vi "Serial_readV1.vi"() -> ()   [LabVIEW 2014]
uses:
  <vilib>/Instr/_visa.llb/VISA Set IO Buffer Mask.ctl
  <vilib>/Instr/_visa.llb/VISA Flush IO Buffer Mask.ctl
  <vilib>/Instr/_visa.llb/VISA Configure Serial Port (Instr).vi
panel:
  out "Svoris 2":cluster{dbl}(graph)
  out "Temperatura":cluster{dbl}(graph)
  in  "Nunulinti":bool
  out "Svoris, N":dbl format="%#_4f"
  out "Svoris":cluster{dbl}(graph)
  out "Svoris, N":dbl(slide) scale=0.0..10000.0
  out "Svoris":dbl
  in  "milliseconds to wait":u32=200
  out "Svoris":dbl(knob) scale=0.0..3.3
  in  "stop":bool
  in  "VISA resource name":refnum<visa-resource-name>
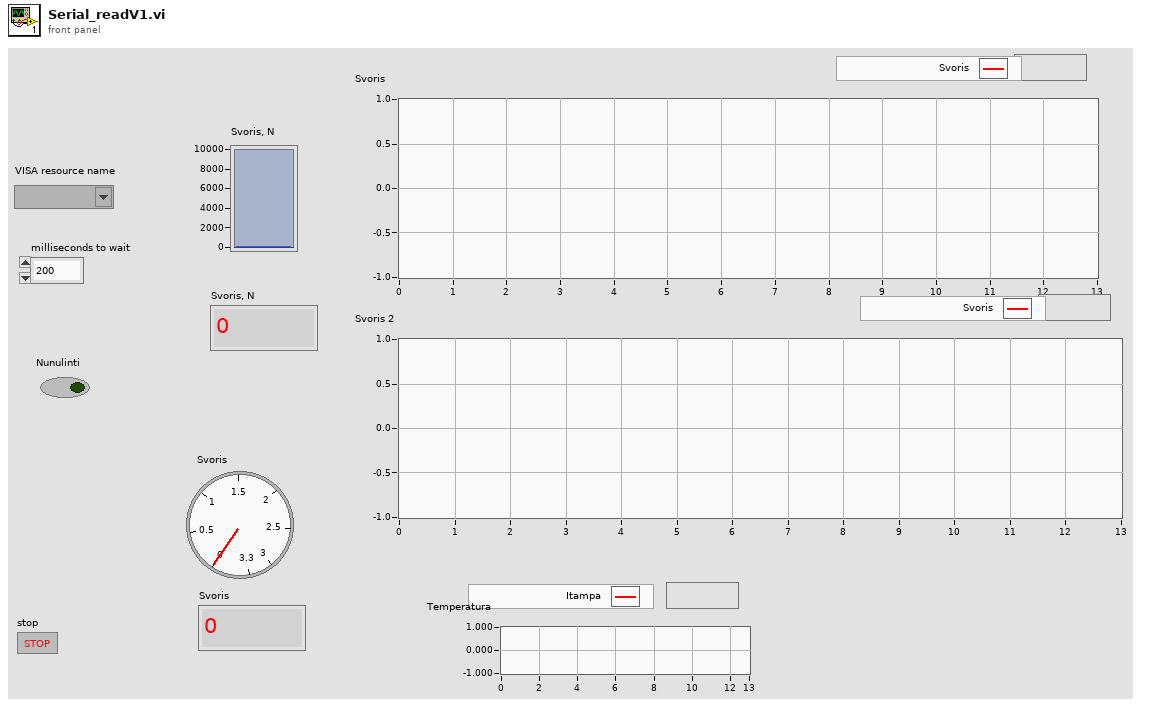
[diagram p1: front panel]
types:
  T1 = typedef "VISA Set IO Buffer Mask.ctl" = u16
  T2 = typedef "VISA Flush IO Buffer Mask.ctl" = u16
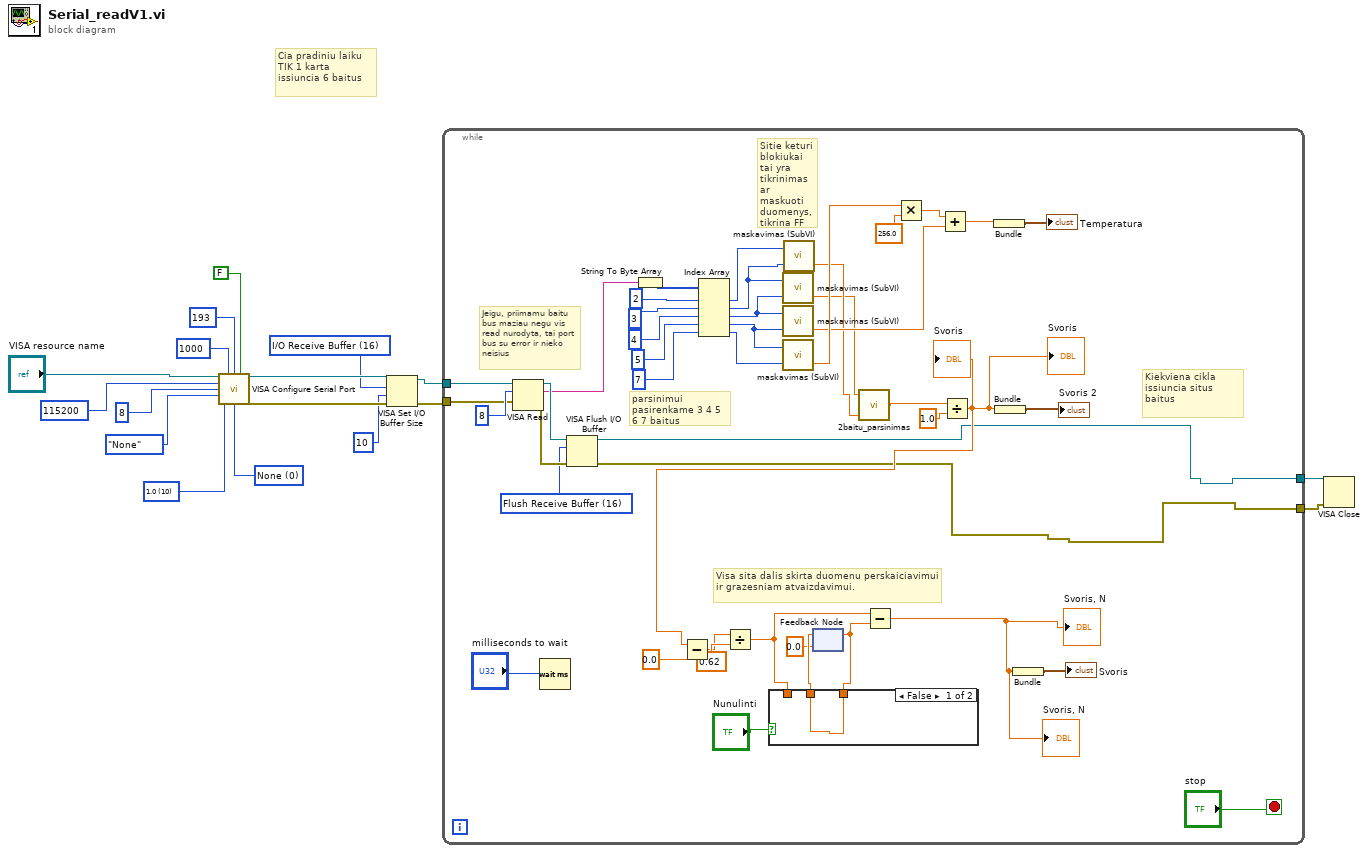
[diagram p0: block diagram]
diagram:
  w7 = T1 16 items=["I/O Receive Buffer"=16, "I/O Transmit Buffer"=32, "I/O Receive and Transmit Buffer"=48] ("Mask")
  w13 = u16 0 items=["None", "XON/XOFF", "RTS/CTS", "XON/XOFF & RTS/CTS", "DTR/DSR", "XON/XOFF & DTR/DSR"] ("flow control (0:none)")
  w14 = u16 10 items=["1.0"=10, "1.5"=15, "2.0"=20] ("stop bits (10: 1 bit)")
  # "Cia pradiniu laiku TIK 1 karta issiuncia 6 baitus"
  n1 = call-poly "VISA Configure Serial Port"("VISA resource name"="VISA resource name", "timeout (10sec)"=u32 1000, "termination char\n(0xA = '\\n' = LF)"=u8 193 ("termination char\n(0xA = '\\n' = LF)"), "Enable Termination\nChar (T)"=FALSE ("Enable Termination\nChar (T)"), "baud rate (9600)"=u32 115200, "data bits (8)"=u16 8, "parity (0:none)"=enum16{"None", "Odd", "Even", "Mark", "Space"}."None", "stop bits (10: 1 bit)"=w14, "flow control (0:none)"=w13) -> ("VISA resource name out"=w9:refnum<visa-resource-name>, "error out"=w10:errorcluster)  [unwired: 5 in]
  n2 = VISA Set I/O Buffer Size(VISA resource name=w9, mask (16)=w7, size (4096)=u32 10, error in (no error)=w10) -> (VISA resource name out=w3:refnum<visa-resource-name>, error out=w6:errorcluster)
  n3 = while {
    tunnel: w3 -> [w61]
    tunnel: w6 -> [w56]
    tunnel: [w19] -> w2
    tunnel: [w18] -> w1
    stop <- "stop" stop-if-true
    w51 = T2 16 items=["Flush Receive Buffer"=16, "Write Transmit Buffer to Device"=32, "Flush Receive Buffer (No I/O)"=64, "Flush Transmit Buffer"=128] ("Mask")
    # "Visa sita dalis skirta duomenu perskaiciavimui ir grazesniam atvaizdavimui."
    # "parsinimui pasirenkame 3 4 5 6 7 baitus"
    # "Sitie keturi blokiukai tai yra tikrinimas ar maskuoti duomenys, tikrina FF"
    # "Kiekviena cikla issiuncia situs baitus"
    # "Jeigu, priimamu baitu bus maziau negu vis read nurodyta, tai port bus su error ir nieko neisius"
    n4 = VISA Read(VISA resource name=w61, byte count=u32 8, error in (no error)=w56) -> (VISA resource name out=w53:refnum<visa-resource-name>, read buffer=w37:string, error out=w52:errorcluster)  [unwired: 1 out]
    n5 = Wait (ms)(milliseconds to wait="milliseconds to wait") -> ()  [unwired: 1 out]
    n6 = VISA Flush I/O Buffer(VISA resource name=w53, mask (16)=w51, error in (no error)=w52) -> (VISA resource name out=w19:refnum<visa-resource-name>, error out=w18:errorcluster)
    n7 = String To Byte Array(string=w37) -> (unsigned byte array=w57:u8[])
    n8 = Index Array "Index Array"(array=w57, index #1=2 ("index"), index #2=3 ("index"), index #3=4 ("index"), index #4=5 ("index"), index #5=7 ("index")) -> (element #1=w36:u8, element #2=w35:u8, element #3=w32:u8, element #4=w31:u8, element #5=w33:u8)
    n9 = call "maskavimas (SubVI).vi"("Numeric 2"=w32, "Numeric"=w35) -> ("Numeric 3"=w22:dbl)  [unwired: 1 in]
    n10 = call "maskavimas (SubVI).vi"("Numeric 2"=w31, "Numeric"=w32) -> ("Numeric 3"=w26:dbl)  [unwired: 1 in]
    n11 = call "maskavimas (SubVI).vi"("Numeric 2"=w33, "Numeric"=w31) -> ("Numeric 3"=w27:dbl)  [unwired: 1 in]
    n12 = call "maskavimas (SubVI).vi"("Numeric 2"=w35, "Numeric"=w36) -> ("Numeric 3"=w23:dbl)  [unwired: 1 in]
    n13 = feedback #1(0.0) -> (w43:dbl)
    n14 = call "2baitu_parsinimas.vi"("Numeric 2"=w23, "Numeric"=w22) -> ("Numeric 3"=w21:dbl)  [unwired: 3 in]
    n15 = Multiply(x=w27, y=256.0) -> (x*y=w25:dbl)
    n16 = Add(x=w25, y=w26) -> (x+y=w28:dbl)
    n17 = Divide(x=w21, y=1.0) -> (x/y=w20:dbl)
    "Svoris" <- w20
    "Svoris" <- w20
    n18 = Subtract(x=w20, y=0.0 ("x")) -> (x-y=w41:dbl)
    n19 = Divide(x=w41, y=0.62) -> (x/y=w42:dbl)
    n20 = case shown="False" "Nunulinti" {
      tunnel: [w62 w63] -> w47
      tunnel: w42 -> [_ w63]
      tunnel: w43 -> [w62 _]
      frame False {
      }
      frame True {
      }
    }
    n21 = feedback-in #1(w47) -> ()
    n22 = Subtract(x=w42, y=w43) -> (x-y=w44:dbl)
    "Svoris, N" <- w44
    "Svoris, N" <- w44
    n23 = Bundle(w28) -> (→"Temperatura":cluster{dbl})  [unwired: 1 in]
    n24 = Bundle(w20) -> (→"Svoris 2":cluster{dbl})  [unwired: 1 in]
    n25 = Bundle(w44) -> (→"Svoris":cluster{dbl})  [unwired: 1 in]
  }
  n26 = VISA Close(VISA resource name=w2, error in (no error)=w1) -> ()  [unwired: 1 out]
